vi "Outlook_Mail_COVID_2019.vi"(4 "BCC":string, 5 "Report Path":path, 6 "CC":string, 7 "Importance":i32(ring)=1 items=["Low", "Normal", "High"], 8 "error in":errorcluster, 9 "Message":string, 10 "Subject":string, 11 "To":string) -> (0 "error out":errorcluster)   [LabVIEW 2019]
doc: "This example uses Microsoft Outlook activeX objects to create a new message and then send that message using the Microsoft Outlook engine. The VI was developed and testing using Microsoft Outlook 2002, but most version of Microsoft Outlook should be compatible with the program.\n\nEnter data into the To, Subject, and message controls on the front panel. The other controls, CC and BCC, are optional. When using multiple email addresses separate addresses with a semicolon. \n\nRun the VI to send an email to the specified email address. If you have the E-mail security update installed with Microsoft Outlook 2002, you will be prompted to authorize the automated email and override the security warning. Click OK in the message box to send the email.\n\nNote: \nFor truly automated messaging, you can override this warning message programmatically using third party software."
panel:
  # "Select Help»Show Context Help and move the cursor over the VI icon to display help for this VI."
  # "Sending E-Mail with MS Outlook Using ActiveX"
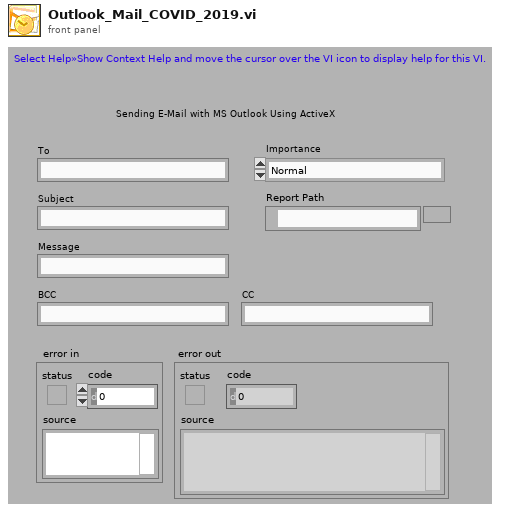
[diagram p1: front panel]
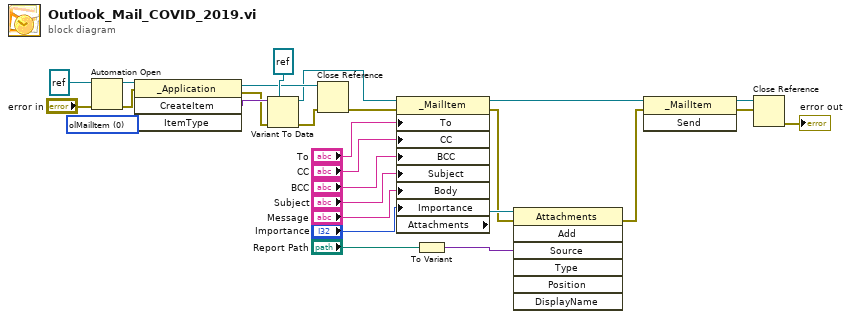
[diagram p0: block diagram]
diagram:
  w25 = 0 items=["olMailItem", "olAppointmentItem", "olContactItem", "olTaskItem", "olJournalItem", "olNoteItem", "olPostItem"] ("ItemType")
  n1 = Automation Open(error in (no error)="error in", Automation Refnum=refnum<k7> refnum ("Outlook._Application")) -> (Automation Refnum=w26:refnum<k7>, error out=w18:errorcluster)  [unwired: 2 in]
  n2 = invoke class="_Application" method="CreateItem"(reference=w26, error in=w18, "ItemType"=w25) -> (reference out=w21:refnum<k7>, error out=w16:errorcluster, "CreateItem"=w24:variant)  [unwired: 1 in, 1 out]
  n3 = Variant To Data(error in=w16, type=refnum<k7> refnum ("Outlook._MailItem"), Variant=w24) -> (data=w1:refnum<k7>, error out=w15:errorcluster)
  n4 = Close Reference(reference=w21, error in (no error)=w15) -> (error out=w14:errorcluster)
  n5 = property class="_MailItem"(reference=w1, error in=w14, "To"="To", "CC"="CC", "BCC"="BCC", "Subject"="Subject", "Body"="Message", "Importance"="Importance") -> (reference out=w2:refnum<k7>, error out=w6:errorcluster, "Attachments"=w7:refnum<k7>)
  n6 = To Variant(anything="Report Path") -> (Variant=w4:variant)
  n7 = invoke class="Attachments" method="Add"(reference=w7, error in=w6, "Source"=w4) -> (error out=w3:errorcluster)  [unwired: 4 in, 6 out]
  n8 = invoke class="_MailItem" method="Send"(reference=w2, error in=w3) -> (reference out=w20:refnum<k7>, error out=w19:errorcluster)  [unwired: 1 in, 1 out]
  n9 = Close Reference(reference=w20, error in (no error)=w19) -> (error out=→"error out":errorcluster)
